vi "GetDevice.vi"(8 "error in (no error)":errorcluster) -> (0 "error out":errorcluster, 1 "found":bool, 3 "device configuration":T1)   [LabVIEW 2017, in "GlobalConfiguration.lvlib"]
uses:
  <vilib>/addons/InsightCM/Utilities/GlobalConfiguration/GlobalConfiguration.lvlib
  <vilib>/addons/InsightCM/MessageBus/Base/controls/R2_Device.ctl
  <vilib>/addons/InsightCM/MessageBus/Base/controls/KeyValuePair.ctl
  <vilib>/addons/InsightCM/MessageBus/Base/controls/DeviceState.ctl
  <vilib>/addons/InsightCM/MessageBus/Base/controls/R2_DataGroup.ctl
  <vilib>/addons/InsightCM/MessageBus/Base/controls/OperatingState.ctl
  <vilib>/addons/InsightCM/MessageBus/Base/controls/Trigger.ctl
  <vilib>/addons/InsightCM/MessageBus/Base/controls/Condition.ctl
  <vilib>/addons/InsightCM/MessageBus/Base/controls/BurstModeTrigger.ctl
  <vilib>/addons/InsightCM/MessageBus/Base/controls/SensorGroup.ctl
  <vilib>/addons/InsightCM/MessageBus/Base/controls/Endpoint.ctl
  <vilib>/addons/InsightCM/MessageBus/Base/controls/WirelessChannel.ctl
  <vilib>/addons/PointValueMap/subVIs/Point_Read_variant.vi
  <vilib>/addons/PointValueMap/subVIs/Point_Write_variant.vi
  <vilib>/addons/PointValueMap/PointValueMap.lvlib
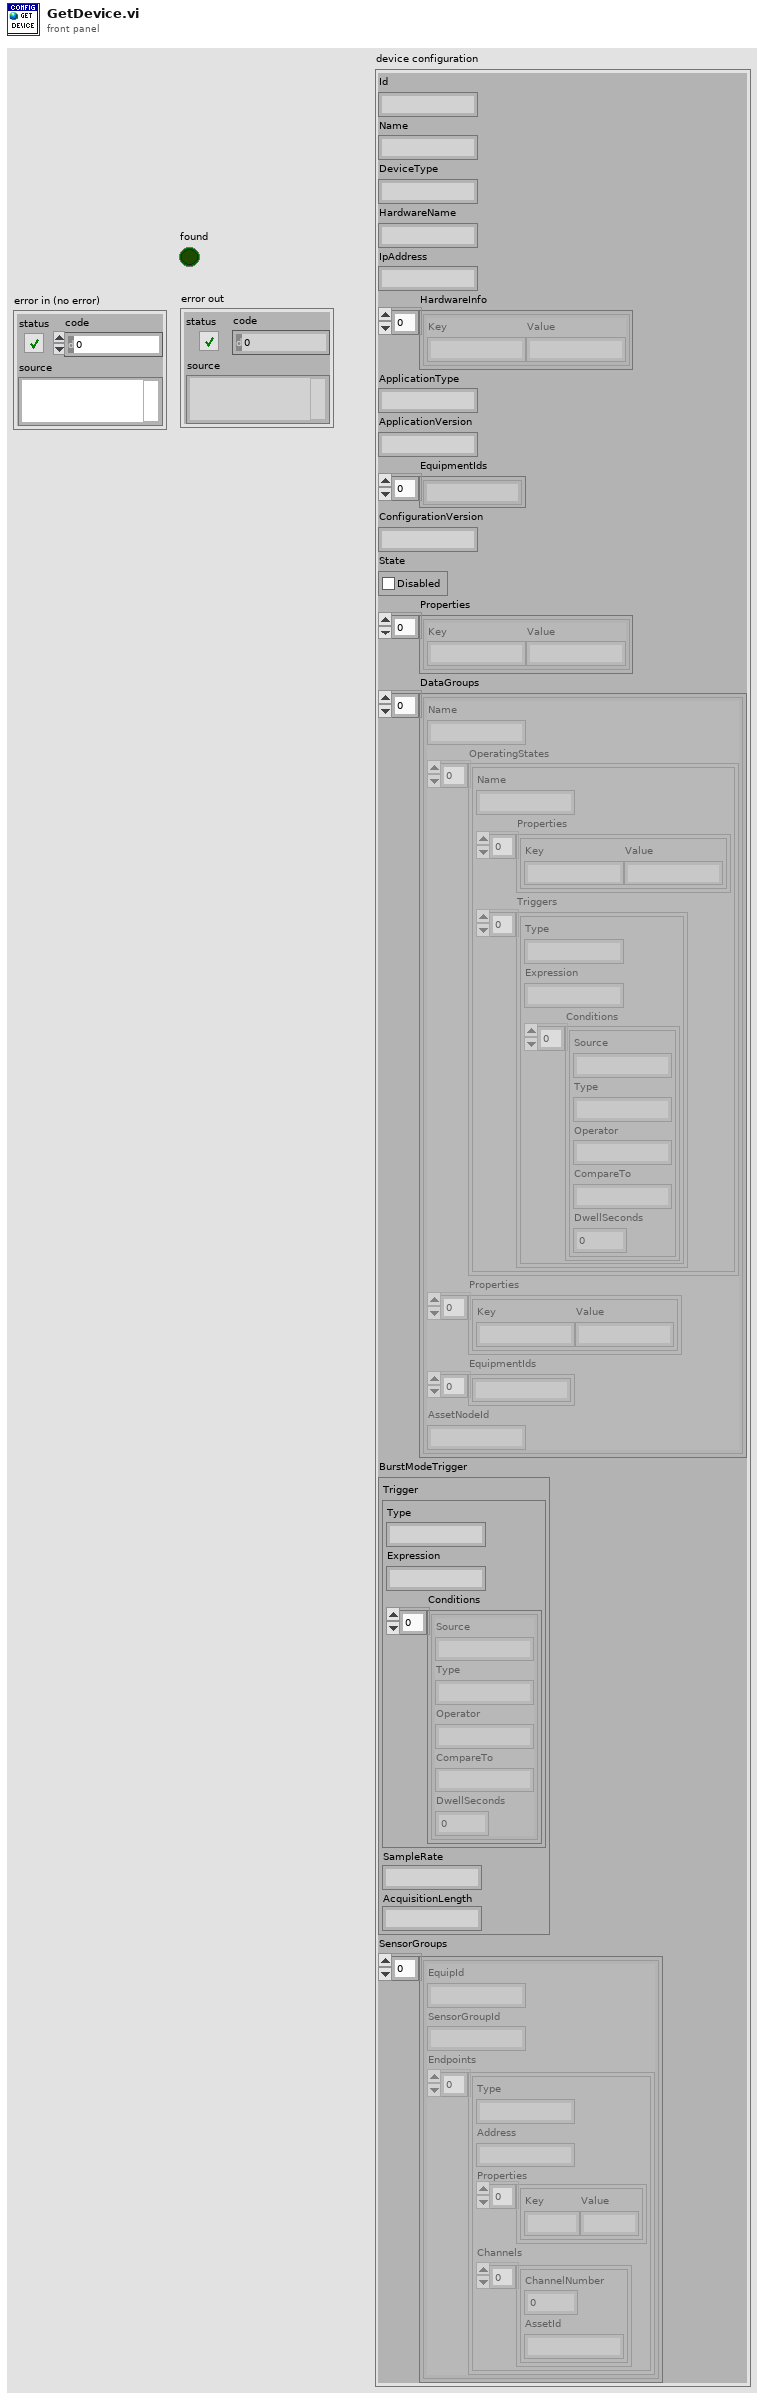
[diagram p1: front panel]
types:
  T1 = typedef "R2_Device.ctl" = cluster{"Id":string, "Name":string, "DeviceType":string, "HardwareName":string, "IpAddress":string, "HardwareInfo":T2[], "ApplicationType":string, "ApplicationVersion":string, "EquipmentIds":string[], "ConfigurationVersion":string, "State":T3, "Properties":T2[], "DataGroups":T4[], "BurstModeTrigger":T8, "SensorGroups":T9[]}
  T2 = typedef "KeyValuePair.ctl" = cluster{"Key":string, "Value":string}
  T3 = typedef "DeviceState.ctl" = cluster{"Disabled":bool}
  T4 = typedef "R2_DataGroup.ctl" = cluster{"Name":string, "OperatingStates":T5[], "Properties":T2[], "EquipmentIds":string[], "AssetNodeId":string}
  T5 = typedef "OperatingState.ctl" = cluster{"Name":string, "Properties":T2[], "Triggers":T6[]}
  T6 = typedef "Trigger.ctl" = cluster{"Type":string, "Expression":string, "Conditions":T7[]}
  T7 = typedef "Condition.ctl" = cluster{"Source":string, "Type":string, "Operator":string, "CompareTo":string, "DwellSeconds":dbl}
  T8 = typedef "BurstModeTrigger.ctl" = cluster{"Trigger":T6, "SampleRate":string, "AcquisitionLength":string}
  T9 = typedef "SensorGroup.ctl" = cluster{"EquipId":string, "SensorGroupId":string, "Endpoints":T10[]}
  T10 = typedef "Endpoint.ctl" = cluster{"Type":string, "Address":string, "Properties":T2[], "Channels":T11[]}
  T11 = typedef "WirelessChannel.ctl" = cluster{"ChannelNumber":i32, "AssetId":string}
  T12 = typedef "PointValueMap.lvlib/PointMap.ctl" = refnum<data-value>
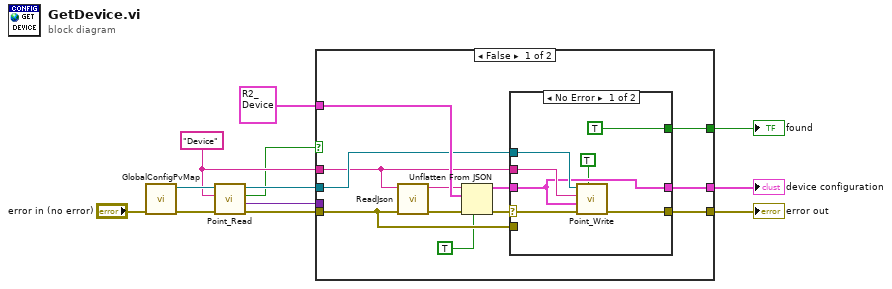
[diagram p0: block diagram]
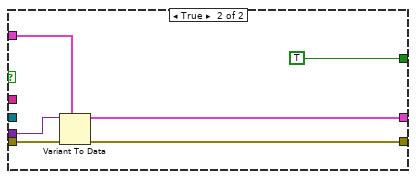
[diagram p3: hidden frame]
diagram:
  w6 = "Device" ("Name")
  n1 = call <vilib>:"GlobalConfigPvMap.vi"("error in (no error)"="error in (no error)") -> ("error out"=w8:errorcluster, "global configuration map"=w9:T12)  [unwired: 9 in]
  n2 = call-poly <vilib>:"Point_Read.vi"("Error In"=w8, "Tag"=w6, "Map"=w9) -> ("Error Out"=w2:errorcluster, "Value"=w3:variant, "Found?"=w1:bool, "Map Out"=w4:T12)  [unwired: 3 in, 2 out]
  n3 = case shown="False" w1 {
    tunnel: [w15 w38] -> w12
    tunnel: [w16 w37] -> w11
    tunnel: [w20 TRUE] -> w7
    tunnel: w6 -> [w18 _]
    tunnel: T1 {"Id"="", "Name"="", "DeviceType"="", "HardwareName"="", "IpAddress"="", "HardwareInfo"=[], "ApplicationType"="", "ApplicationVersion"="", "EquipmentIds"=[], "ConfigurationVersion"="", "State"={"Disabled"=FALSE}, "Properties"=[], "DataGroups"=[], "BurstModeTrigger"={"Trigger"={"Type"="", "Expression"="", "Conditions"=[]}, "SampleRate"="", "AcquisitionLength"=""}, "SensorGroups"=[]} ("Device") -> [w23 w35]
    tunnel: w4 -> [w19 _]
    tunnel: w3 -> [_ w34]
    tunnel: w2 -> [w14 w33]
    frame False {
      n4 = call <vilib>:"ReadJson.vi"("error in (no error)"=w14, "json object"=w18) -> ("error out"=w24:errorcluster, "json string"=w22:string)  [unwired: 8 in]
      n5 = Unflatten From JSON(JSON string=w22, type and defaults=w23, default null elements? (F)=TRUE, error in (no error)=w24) -> (value=w17:T1, error out=w21:errorcluster)  [unwired: 3 in]
      n6 = case shown="No Error" w21 {
        selector: w21 -> [w31 _]
        tunnel: [TRUE _] -> w20
        tunnel: w19 -> [w29 _]
        tunnel: w18 -> [w28 _]
        tunnel: w17 -> [w27 _]
        tunnel: [w27 _] -> w16
        tunnel: [w26 w32] -> w15
        tunnel: w14 -> [_ w32]
        frame No Error {
          n7 = call-poly <vilib>:"Point_Write.vi"("Auto Create?"=TRUE, "Error In"=w31, "Value"=w27, "Tag"=w28, "Map"=w29) -> ("Error Out"=w26:errorcluster)  [unwired: 5 in, 1 out]
        }
        frame Error {
        }
      }
    }
    frame True {
      n8 = Variant To Data(error in=w33, type=w35, Variant=w34) -> (data=w37:T1, error out=w38:errorcluster)
    }
  }
  "error out" <- w12
  "device configuration" <- w11
  "found" <- w7
